vi "Set Position and Wait.vi"(8 "error in":errorcluster, 11 "Position":sgl) -> (0 "error out":errorcluster, 3 "Position out":dbl)   [LabVIEW 2019, in "Rotation Stage.lvlib"]
uses:
  Rotation Stage.lvlib
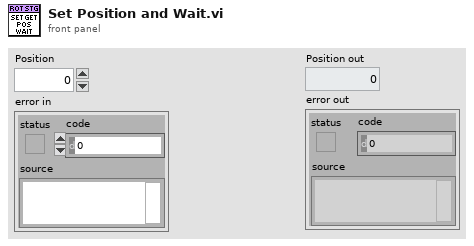
[diagram p1: front panel]
types:
  T1 = typedef "Rotation Stage.lvlib/Get Position (Reply Payload)--cluster.ctl" = cluster{"Position":dbl, "Get Position_error":errorcluster}
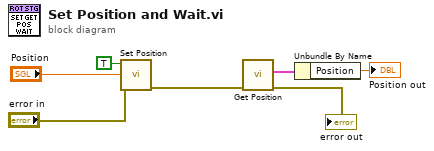
[diagram p0: block diagram]
diagram:
  n1 = call "Set Position.vi"("error in (no error)"="error in", "Position"="Position", "Wait"=TRUE) -> ("error out"=w1:errorcluster)  [unwired: 8 in]
  n2 = call "Get Position.vi"("error in (no error)"=w1) -> ("error out"=→"error out":errorcluster, "Reply Payload"=w5:T1)  [unwired: 8 in, 1 out]
  n3 = Unbundle By Name(w5) -> ("Position"=→"Position out":dbl)
